vi "Regler FT-IR_Ausgang NEU.vi"(7 "Index":i32, 8 "Fehler":errorcluster caption="Fehler (Eingang)") -> (0 "Fehler (Ausgang)":errorcluster)   [LabVIEW 2020, in "Regler.lvlib" / "Druckregler.lvlib"]
uses:
  Druckregler.lvlib
  Aktionen Param. Druckregler.ctl
  Visualisierungs Elemente/Zahlen-Eingabefeld.ctl
  Verwaltung/FGV IN Aktionen.ctl
  Konfig-Dateien/FGV Betriebsdaten Aktionen.ctl
  Allgemein/Aktionen FGV Dichtheitstest.ctl
  Allgemein/Aktion FGV Messbetrieb.ctl
  Aktionen Interne Werte.ctl
  Verwaltung/Verwaltung - cRIO.lvlib
  Allgemein/Allgemein.lvlib
  Konfig-Dateien/Konfig-Dateien.lvlib
  Verwaltung/FGV OUT Aktionen.ctl
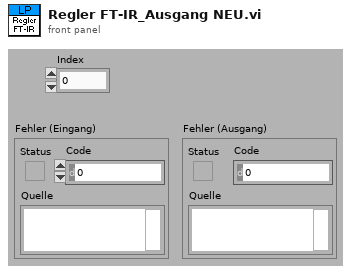
[diagram p1: front panel]
types:
  T1 = typedef "Allgemein.lvlib/Aktion FGV Messbetrieb.ctl" = enum16{"lesen", "schreiben"}
  T2 = typedef "Allgemein.lvlib/Aktionen FGV Dichtheitstest.ctl" = enum16{"lesen", "schreiben"}
  T3 = typedef "Zahlen-Eingabefeld.ctl" = sgl
  T4 = typedef "Konfig-Dateien.lvlib/FGV Betriebsdaten Aktionen.ctl" = enum16{"lesen", "Anlagengrenzw.", "PID Param.", "Sonstige", "Sensor Para."}
  T5 = typedef "Verwaltung - cRIO.lvlib/FGV IN Aktionen.ctl" = enum16{"lesen", "DI", "AI", "Fühler Br.", "TC", "Fühler Br. TC"}
  T6 = typedef "Regler.lvlib/Druckregler.lvlib/Aktionen Param. Druckregler.ctl" = enum16{"lesen", "schreiben", "Regler FT-IR", "Regler Ausgang", "Regler Durchfluss", "Regler PMA", "Regler NDIR", "Regler Filterblock", "Regler Gaskühler", "Regler Kalter Block"}
  T7 = typedef "Anlagengrenzwerte.lvlib/Anlagen-Grenzwerte Anzeige.ctl" = cluster{"Eingangsdruck FT-IR:":T8, "Durchfluss FT-IR:":T8, "Durchfluss CalGas:":T8, "Druck Ausgang:":T8, "Druck Kalter Block:":T8, "Heizleitungen intern:":T8, "Heizleitung zu FT-IR:":T8, "Heizung Filterblock:":T8, "Heizung Pumpe:":T8, "Heizleitung Extern SP1:":T8, "Heizleitung Extern SP2:":T8, "FT-IR Heizung Messzelle:":T8, "Schaltschranktemperatur:":T8, "Gaskühler:":T8}
  T8 = typedef "Anlagengrenzwerte.lvlib/Anlagen-Parameter Anzeige.ctl" = cluster{"Sollwert":sgl, "Warn-Min":sgl, "Warn-Max":sgl, "Abschalt-Min":sgl, "Abschalt-Max":sgl, "Regler":u16}
  T9 = typedef "Verwaltung - cRIO.lvlib/Analog Eingaenge.ctl" = cluster{"AI0: Durchfluss FT-IR":sgl, "AI1: Druck Ausgang":sgl, "AI2: Umgebungsdruck":sgl, "AI3: Druck FT-IR":sgl, "AI4: Druck CalGas":sgl, "AI5: Reserve":sgl, "AI6: Reserve":sgl, "AI7: Reserve":sgl, "Rohwert Durchfluss FT-IR":sgl, "Rohwert Druck Ausgang":sgl, "Rohwert Umgebungsdruck":sgl, "Rohwert Druck FT-IR":sgl, "Rohwert Druck CalGas":sgl, "Rohwert AI5":sgl, "Rohwert AI6":sgl, "Rohwert AI7":sgl, "Rohwert Diffdruck mbar FTIR":sgl}
  T10 = typedef "Verwaltung - cRIO.lvlib/FGV OUT Aktionen.ctl" = enum16{"lesen", "ANA OUT", "DO 0-31", "DO 32-47"}
  T11 = typedef "Regler.lvlib/Druckregler.lvlib/Aktionen Interne Werte.ctl" = enum16{"lesen", "FT-IR", "Ausgang", "Pumpe", "laden", "speichern", "Änderung?", "Druck Kalter Block", "Dichtheitstest"}
  T12 = typedef "Verwaltung - cRIO.lvlib/Analog Eingaenge.ctl" = cluster{"AI0: Durchfluss FT-IR":sgl, "AI1: Druck Ausgang":sgl, "AI2: Umgebungsdruck":sgl, "AI3: Druck FT-IR":sgl, "AI4: Druck CalGas":sgl, "AI5: Reserve":sgl, "AI6: Reserve":sgl, "AI7: Reserve":sgl, "Rohwert Durchfluss FT-IR":sgl, "Rohwert Druck Ausgang":sgl, "Rohwert Umgebungsdruck":sgl, "Rohwert Druck FT-IR":sgl, "Rohwert Durchfluss MW":sgl, "TC0: Schaltschrank":sgl, "TC1: Filterblock":sgl, "TC2: HL intern":sgl, "TC3: HL Extern SP1":sgl, "TC4: Temperatur FTIR":sgl, "TC5: Gastemperatur":sgl, "TC6: Temperatur Extern 1":sgl, "TC7: Temperatur Extern 2":sgl}
  T13 = typedef "Verwaltung - cRIO.lvlib/Digital Ausgaenge 0-31.ctl" = cluster{"O0: Druckluft Versorgung":bool, "O1: CG 1 (FB Eingang 1)":bool, "O2: CG 2 (Kühlung FT-IR EIN)":bool, "O3: CG 3 (FB Bypass)":bool, "O4: CG 4 (FB CalGas)":bool, "O5: CG 5 (FB spülen/UL)":bool, "O6: CG 6 (FB zum FT-IR)":bool, "O7: CG 7 (FB zum FID)":bool, "O8: CG 8 (FB Reserve)":bool, "O9: (FB Reserve)":bool, "O10: (FB Umgebungsluft FID)":bool, "O11: (FB zum Gaskühler)":bool, "O12: FB Stickstoff zu FT-IR":bool, "O13: Optikbox FT-IR spülen":bool, "O14: (Purifier deaktivieren)":bool, "O15: (Umschaltung Purifier/Stickstoff)":bool, "O16: N2 Einblasung":bool, "O17: LSP LN2 Nachfüllung":bool, "O18: (Reserve)":bool, "O19: (Pumpe Eingang1)":bool, "O20: (Pumpe Eingang2)":bool, "O21: (Pumpe Spülen1)":bool, "O22: (Pumpe Spülen2)":bool, "O23: (Reserve)":bool, "O24: CalGas 1":bool, "O25: CalGas 2":bool, "O26: CG 3-8 (CalGas 3)":bool, "O27: Stickstoff aufschalten":bool, "O28: CG zu PNS":bool, "O29: FTIR Standby Spülung":bool, "O30: CG zu Entnahme(T90)":bool, "O31: (Purifier regenerieren)":bool}
  T14 = cluster{"Numerisch":sgl, "Numerisch":sgl, "Numerisch":sgl, "Numerisch":sgl, "Numerisch":sgl}
  T15 = typedef "Regler.lvlib/Druckregler.lvlib/Regler Interne Werte.ctl" = cluster{"PV":sgl, "D-action":sgl, "Error":sgl, "I-action":sgl, "OUT":sgl}
  T16 = typedef "Erweiterte Konfig.lvlib/Aktionen Dichtheitstest.ctl" = enum16{"Initialisieren", "Unterdruck aufbauen", "Prop schließen", "Warten", "Auswertung", "Fertig"}
  T17 = typedef "EPA 1065.lvlib/Dichtheitstest 1065-345.lvlib/Aktion Leak check durchfuehren.ctl" = enum16{"initialisieren", "Unterdruck erzeugen", "Ventile schließen", "Warten", "Auswertung", "fertig", "PDF erstellen", "abbrechen"}
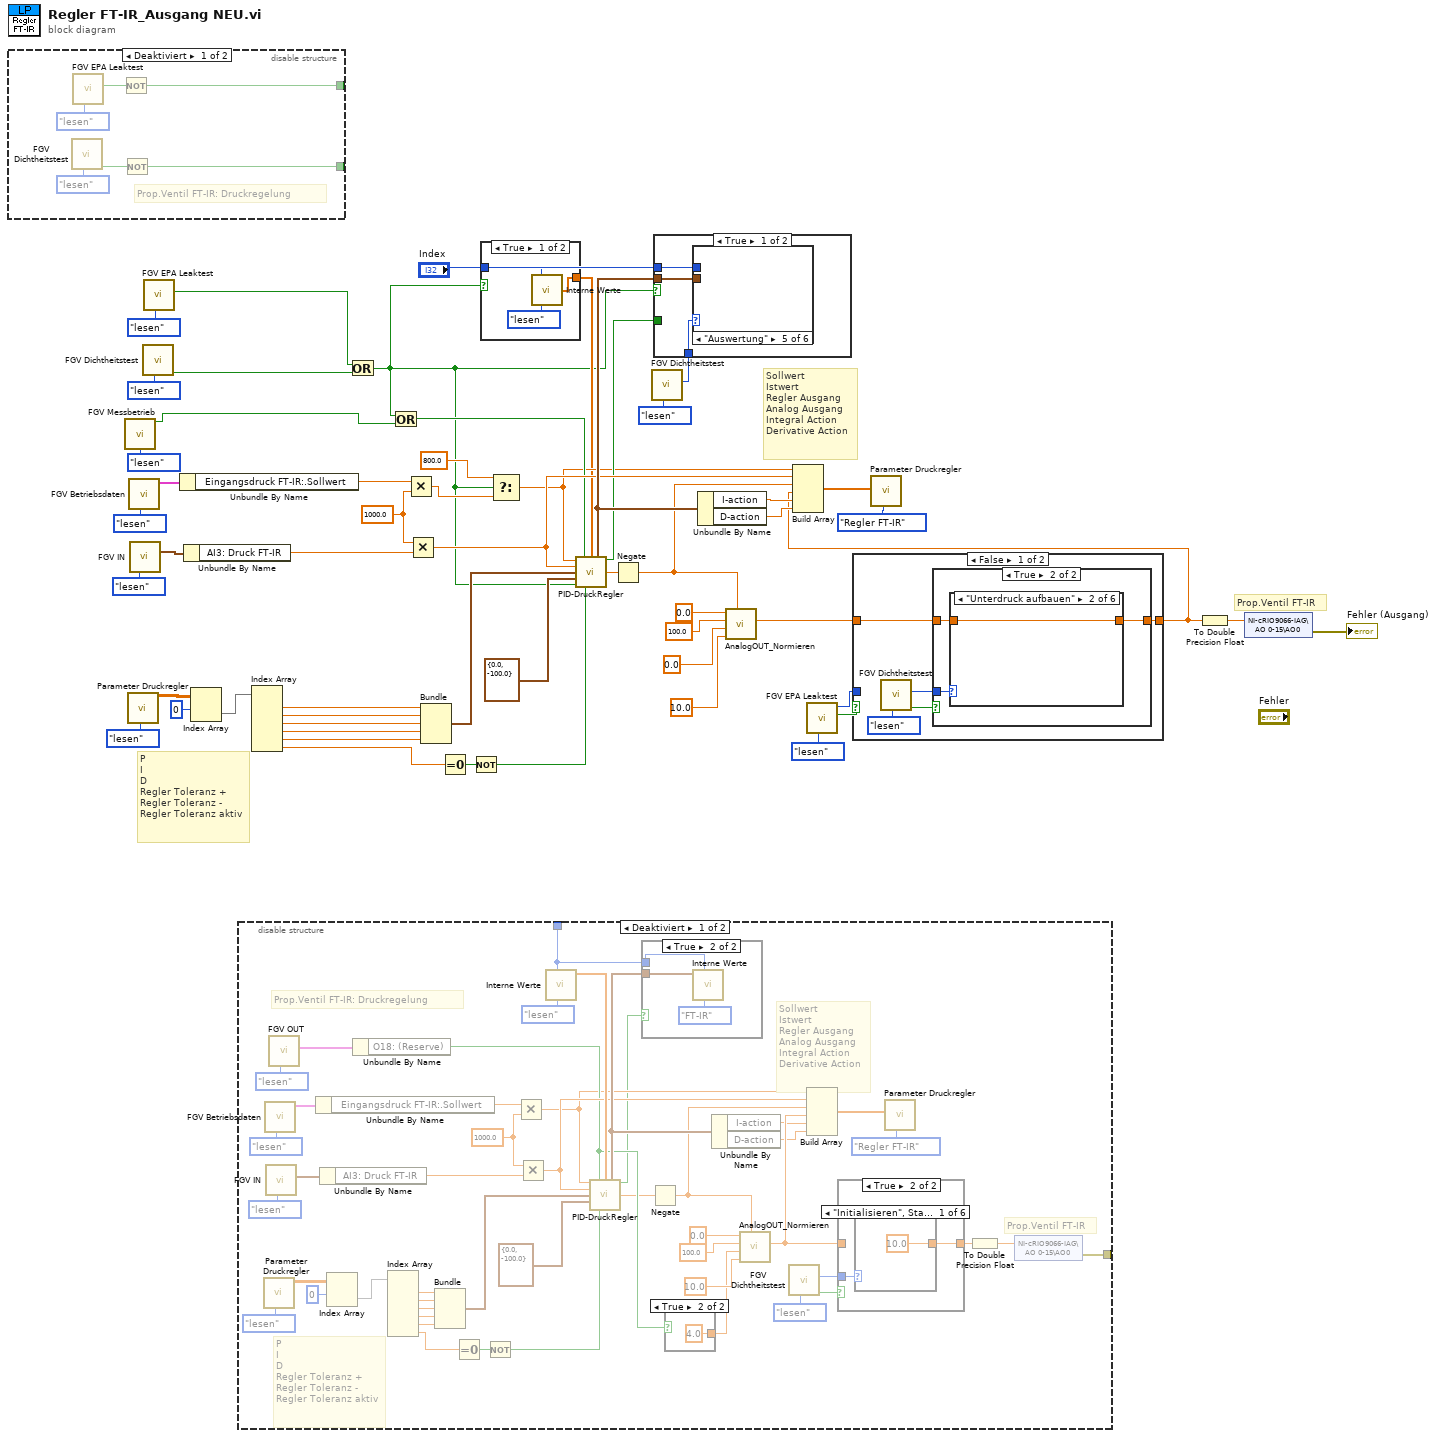
[diagram p0: block diagram]
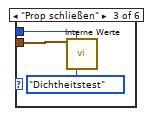
[diagram p4: hidden frame]
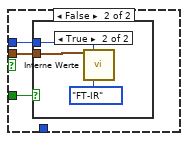
[diagram p7: hidden frame]
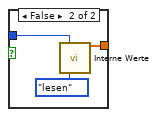
[diagram p9: hidden frame]
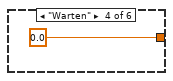
[diagram p13: hidden frame]
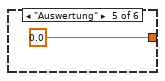
[diagram p14: hidden frame]
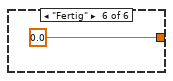
[diagram p15: hidden frame]
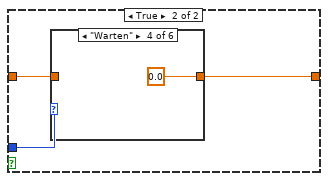
[diagram p16: hidden frame]
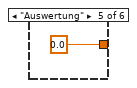
[diagram p20: hidden frame]
diagram:
  w34 = T3 1000.0 ("y")
  # "Prop.Ventil FT-IR"
  # "Sollwert\nIstwert\nRegler Ausgang\nAnalog Ausgang\nIntegral Action\nDerivative Action"
  # "P\nI\nD\nRegler Toleranz +\nRegler Toleranz -\nRegler Toleranz aktiv"
  n1 = disable-structure shown="Deaktiviert" {
    disable-tunnel: [w60 _] -> _
    disable-tunnel: [w57 _] -> _
    frame Disabled {
      # "Prop.Ventil FT-IR: Druckregelung"
      n2 = call "FGV Dichtheitstest.vi"("Aktionen"=Aktionen_FGV_Dichtheitstest."lesen") -> ("Dichtheitstest?"=w61:bool)  [unwired: 9 in, 1 out]
      n3 = call "FGV EPA Leaktest.vi"("Aktion"=enum16{"lesen", "schreiben"}."lesen") -> ("Leaktest aktiv"=w58:bool)  [unwired: 9 in, 1 out]
      n4 = Not(x=w58) -> (.not. x?=w57:bool)
      n5 = Not(x=w61) -> (.not. x?=w60:bool)
    }
    frame Enabled {
    }
  }
  n6 = call "FGV Messbetrieb.vi"("Aktion"=Aktion_FGV_Messbetrieb."lesen") -> ("messen"=w1:bool)  [unwired: 13 in, 1 out]
  n7 = call "Parameter Druckregler.vi"("Aktionen"=Aktionen_Param._Druckregler."lesen") -> ("Regleparameter"=w39:sgl[][])  [unwired: 10 in, 8 out]
  n8 = call "FGV Betriebsdaten.vi"("Aktionen"=FGV_Betriebsdaten_Aktionen."lesen") -> ("Anlagen-Grenzwerte"=w24:T7)  [unwired: 7 in, 3 out]
  n9 = call "FGV IN.vi"("Aktion"=FGV_IN_Aktionen."lesen") -> ("Analog Eingänge"=w23:T9)  [unwired: 10 in, 4 out]
  n10 = call "FGV Dichtheitstest.vi"("Aktionen"=Aktionen_FGV_Dichtheitstest."lesen") -> ("Dichtheitstest?"=w18:bool)  [unwired: 9 in, 1 out]
  n11 = call "FGV EPA Leaktest.vi"("Aktion"=enum16{"lesen", "schreiben"}."lesen") -> ("Leaktest aktiv"=w13:bool)  [unwired: 9 in, 1 out]
  n12 = Unbundle By Name(w24) -> ("Eingangsdruck FT-IR:.Sollwert"=w35:sgl)
  n13 = Unbundle By Name(w23) -> ("AI3: Druck FT-IR"=w33:sgl)
  n14 = Index Array(array=w39, index (row)=0 ("Deaktivierter Index (Spalte)")) -> (element=w38:sgl[])  [unwired: 1 in]
  n15 = disable-structure shown="Deaktiviert" {
    disable-tunnel: _ -> [w73 _]
    disable-tunnel: [w69 _] -> _
    frame Disabled {
      w88 = T3 1000.0 ("y")
      # "Prop.Ventil FT-IR"
      # "Prop.Ventil FT-IR: Druckregelung"
      # "Sollwert\nIstwert\nRegler Ausgang\nAnalog Ausgang\nIntegral Action\nDerivative Action"
      # "P\nI\nD\nRegler Toleranz +\nRegler Toleranz -\nRegler Toleranz aktiv"
      n16 = call "Parameter Druckregler.vi"("Aktionen"=Aktionen_Param._Druckregler."lesen") -> ("Regleparameter"=w93:sgl[][])  [unwired: 7 in, 3 out]
      n17 = call "FGV Betriebsdaten.vi"("Aktionen"=FGV_Betriebsdaten_Aktionen."lesen") -> ("Anlagen-Grenzwerte"=w64:T7)  [unwired: 7 in, 3 out]
      n18 = call "FGV IN.vi"("Aktion"=FGV_IN_Aktionen."lesen") -> ("Analog Eingänge"=w63:T12)  [unwired: 8 in, 2 out]
      n19 = call "FGV OUT.vi"("Aktion"=FGV_OUT_Aktionen."lesen") -> ("DO 0-31"=w65:T13)  [unwired: 7 in, 3 out]
      n20 = Unbundle By Name(w64) -> ("Eingangsdruck FT-IR:.Sollwert"=w89:sgl)
      n21 = Unbundle By Name(w63) -> ("AI3: Druck FT-IR"=w87:sgl)
      n22 = Index Array(array=w93, index (row)=0 ("Deaktivierter Index (Spalte)")) -> (element=w92:sgl[])  [unwired: 1 in]
      n23 = Unbundle By Name(w65) -> ("O18: (Reserve)"=w78:bool)
      n24 = Index Array(array=w92) -> (element #1=w104:sgl, element #2=w103:sgl, element #3=w102:sgl, element #4=w101:sgl, element #5=w100:sgl, element #6=w75:sgl)  [unwired: 6 in]
      n25 = Bundle("Numerisch"=w104, "Numerisch"=w103, "Numerisch"=w102, "Numerisch"=w101, "Numerisch"=w100) -> (w98:T14)  [unwired: 1 in]
      n26 = Equal To 0?(x=w75) -> (x = 0?=w99:bool)
      n27 = Not(x=w99) -> (.not. x?=w97:bool)
      n28 = Multiply(x=w89, y=w88) -> (x*y=w77:T3)
      n29 = Multiply(x=w88, y=w87) -> (x*y=w86:T3)
      n30 = call "Interne Werte.vi"("Aktionen Interne Werte"=Aktionen_Interne_Werte."lesen", "Index"=w73) -> ("FT-IR"=w110:sgl[])  [unwired: 4 in, 5 out]
      n31 = call "PID-DruckRegler.vi"("Sollwert"=w77, "Regler EIN"=w78, "Regler Interne Werte"=w110, "Istwert"=w86, "PID-Parameter"=w98, "output range"=cluster{"output high":dbl, "output low":dbl} {"output high"=0.0, "output low"=-100.0}, "Regler Toleranz verwenden?"=w97) -> ("Regler Interne Werte"=w109:T15, "Interne Werte speichern"=w72:bool, "Output"=w76:sgl)  [unwired: 6 in]
      n32 = case shown="True" w72 {
        tunnel: w73 -> [_ w112]
        tunnel: w109 -> [_ w111]
        frame False {
        }
        frame True {
          n33 = call "Interne Werte.vi"("Aktionen Interne Werte"=Aktionen_Interne_Werte."FT-IR", "Index"=w112, "Regler Interne Werte"=w111) -> ()  [unwired: 3 in, 6 out]
        }
      }
      n34 = Negate(x=w76) -> (-x=w79:sgl)
      n35 = case shown="True" w78 {
        tunnel: [sgl 0.0 ("Untergrenze") sgl 4.0 ("Untergrenze")] -> w96
        frame False {
        }
        frame True {
        }
      }
      n36 = Unbundle By Name(w109) -> ("I-action"=w71:sgl, "D-action"=w70:sgl)
      n37 = call "AnalogOUT_Normieren.vi"("Analogwert"=w79, "Obergrenze"=sgl 10.0, "Untergrenze"=w96, "Max Analogwert"=sgl 100.0, "Min Analogwert"=sgl 0.0) -> ("Normierter Wert"=w83:sgl)  [unwired: 6 in]
      n38 = call "FGV Dichtheitstest.vi"("Aktionen"=Aktionen_FGV_Dichtheitstest."lesen") -> ("Dichtheitstest?"=w80:bool, "Aktionen Dichtheitstest"=w81:T16)  [unwired: 9 in]
      n39 = Build Array(w77, w86, w79, w83, w71, w70) -> (w91:T3[])
      n40 = case shown="True" w80 {
        tunnel: w81 -> [_ w116]
        tunnel: w83 -> [w114 _]
        tunnel: [w114 w115] -> w82
        frame False {
        }
        frame True {
          n41 = case shown="\"Initialisieren\", Standard" w116 {
            tunnel: [sgl 10.0 ("Untergrenze") sgl 10.0 ("Untergrenze") sgl 0.0 ("Untergrenze") sgl 0.0 ("Untergrenze") sgl 0.0 ("Untergrenze") sgl 0.0 ("Untergrenze")] -> w115
            frame "Initialisieren", Default {
            }
            frame "Unterdruck aufbauen" {
            }
            frame "Warten" {
            }
            frame "Prop schließen" {
            }
            frame "Auswertung" {
            }
            frame "Fertig" {
            }
          }
        }
      }
      n42 = call "Parameter Druckregler.vi"("Aktionen"=Aktionen_Param._Druckregler."Regler FT-IR", "Werte FT-IR"=w91) -> ()  [unwired: 6 in, 4 out]
      n43 = To Double Precision Float(number=w82) -> (double precision float=w85:dbl)
      n44 = shared-variable "NI-cRIO9066-IAG\\AO 0-15\\AO0"(w85) -> (error out=w69:errorcluster)  [unwired: 1 in]
    }
    frame Enabled {
    }
  }
  n45 = Index Array(array=w38) -> (element #1=w50:sgl, element #2=w49:sgl, element #3=w48:sgl, element #4=w47:sgl, element #5=w46:sgl, element #6=w30:sgl)  [unwired: 6 in]
  n46 = Or(x=w13, y=w18) -> (x .or. y?=w3:bool)
  n47 = Or(x=w3, y=w1) -> (x .or. y?=w19:bool)
  n48 = Multiply(x=w35, y=w34) -> (x*y=w17:T3)
  n49 = Multiply(x=w34, y=w33) -> (x*y=w32:T3)
  n50 = Bundle("Numerisch"=w50, "Numerisch"=w49, "Numerisch"=w48, "Numerisch"=w47, "Numerisch"=w46) -> (w44:T14)  [unwired: 1 in]
  n51 = Equal To 0?(x=w30) -> (x = 0?=w45:bool)
  n52 = Not(x=w45) -> (.not. x?=w43:bool)
  n53 = case shown="True" w3 {
    tunnel: "Index" -> [w127 w130]
    tunnel: [w125 w128] -> w6
    frame True {
      n54 = call "Interne Werte.vi"("Index"=w127, "Aktionen Interne Werte"=Aktionen_Interne_Werte."lesen") -> ("Dichtheitstest"=w125:sgl[])  [unwired: 7 in, 6 out]
    }
    frame False {
      n55 = call "Interne Werte.vi"("Index"=w130, "Aktionen Interne Werte"=Aktionen_Interne_Werte."lesen") -> ("FT-IR"=w128:sgl[])  [unwired: 7 in, 6 out]
    }
  }
  n56 = Select(t=T3 800.0, s=w3, f=w17) -> (s? t:f=w15:T3)
  n57 = call "PID-DruckRegler.vi"("Sollwert"=w15, "Regler EIN"=w19, "Regler Interne Werte"=w6, "Istwert"=w32, "PID-Parameter"=w44, "output range"=cluster{"output high":dbl, "output low":dbl} {"output high"=0.0, "output low"=-100.0}, "Dichtheitstest"=w3, "Regler Toleranz verwenden?"=w43) -> ("Regler Interne Werte"=w55:T15, "Interne Werte speichern"=w29:bool, "Output"=w22:sgl)  [unwired: 5 in]
  n58 = Negate(x=w22) -> (-x=w21:sgl)
  n59 = call "FGV Dichtheitstest.vi"("Aktionen"=Aktionen_FGV_Dichtheitstest."lesen") -> ("Aktionen Dichtheitstest"=w4:T16)  [unwired: 9 in, 1 out]
  n60 = case shown="True" w3 {
    tunnel: w55 -> [w133 w139]
    tunnel: w29 -> [_ w138]
    tunnel: "Index" -> [w132 w137]
    tunnel: w4 -> [w131 _]
    frame True {
      n61 = case shown="\"Auswertung\"" w131 {
        tunnel: w132 -> [_ _ w135 _ _ _]
        tunnel: w133 -> [_ _ w134 _ _ _]
        frame "Initialisieren", Default {
        }
        frame "Unterdruck aufbauen" {
        }
        frame "Prop schließen" {
          n62 = call "Interne Werte.vi"("Regler Interne Werte"=w134, "Index"=w135, "Aktionen Interne Werte"=Aktionen_Interne_Werte."Dichtheitstest") -> ()  [unwired: 6 in, 7 out]
        }
        frame "Warten" {
        }
        frame "Auswertung" {
        }
        frame "Fertig" {
        }
      }
    }
    frame False {
      n63 = case shown="True" w138 {
        tunnel: w137 -> [_ w141]
        tunnel: w139 -> [_ w140]
        frame False {
        }
        frame True {
          n64 = call "Interne Werte.vi"("Regler Interne Werte"=w140, "Index"=w141, "Aktionen Interne Werte"=Aktionen_Interne_Werte."FT-IR") -> ()  [unwired: 6 in, 7 out]
        }
      }
    }
  }
  n65 = Unbundle By Name(w55) -> ("I-action"=w28:sgl, "D-action"=w27:sgl)
  n66 = call "AnalogOUT_Normieren.vi"("Analogwert"=w21, "Obergrenze"=sgl 10.0, "Untergrenze"=sgl 0.0, "Max Analogwert"=sgl 100.0, "Min Analogwert"=sgl 0.0) -> ("Normierter Wert"=w9:sgl)  [unwired: 6 in]
  n67 = call "FGV EPA Leaktest.vi"("Aktion"=enum16{"lesen", "schreiben"}."lesen") -> ("Leaktest aktiv"=w11:bool, "Leaktest Zustand"=w10:T17)  [unwired: 9 in]
  n68 = case shown="False" w11 {
    tunnel: w9 -> [w147 w158]
    tunnel: [w146 w160] -> w8
    tunnel: w10 -> [_ w159]
    frame False {
      n69 = call "FGV Dichtheitstest.vi"("Aktionen"=Aktionen_FGV_Dichtheitstest."lesen") -> ("Dichtheitstest?"=w143:bool, "Aktionen Dichtheitstest"=w144:T16)  [unwired: 9 in]
      n70 = case shown="True" w143 {
        tunnel: w144 -> [_ w151]
        tunnel: w147 -> [w148 w149]
        tunnel: [w148 w150] -> w146
        frame False {
        }
        frame True {
          n71 = case shown="\"Unterdruck aufbauen\"" w151 {
            tunnel: [w152 w153 w154 sgl 0.0 ("Untergrenze") sgl 0.0 ("Untergrenze") sgl 0.0 ("Untergrenze")] -> w150
            tunnel: w149 -> [w152 w153 w154 _ _ _]
            frame "Initialisieren", Default {
            }
            frame "Unterdruck aufbauen" {
            }
            frame "Prop schließen" {
            }
            frame "Warten" {
            }
            frame "Auswertung" {
            }
            frame "Fertig" {
            }
          }
        }
      }
    }
    frame True {
      n72 = case shown="\"Warten\"" w159 {
        tunnel: [w161 w162 w163 sgl 0.0 ("Untergrenze") sgl 0.0 ("Untergrenze") sgl 0.0 ("Untergrenze")] -> w160
        tunnel: w158 -> [w161 w162 w163 _ _ _]
        frame "initialisieren", Default {
        }
        frame "Unterdruck erzeugen" {
        }
        frame "Ventile schließen" {
        }
        frame "Warten" {
        }
        frame "Auswertung" {
        }
        frame "fertig" {
        }
      }
    }
  }
  n73 = Build Array(w15, w32, w21, w8, w28, w27) -> (w37:T3[])
  n74 = call "Parameter Druckregler.vi"("Werte FT-IR"=w37, "Aktionen"=Aktionen_Param._Druckregler."Regler FT-IR") -> ()  [unwired: 9 in, 9 out]
  n75 = To Double Precision Float(number=w8) -> (double precision float=w31:dbl)
  n76 = shared-variable "NI-cRIO9066-IAG\\AO 0-15\\AO0"(w31) -> (error out=→"Fehler (Ausgang)":errorcluster)  [unwired: 1 in]
